vi "_27_Sample_qsns_9[3].vi"() -> ()   [LabVIEW 2020]
panel:
  out "Array":i32[](array[numeric])
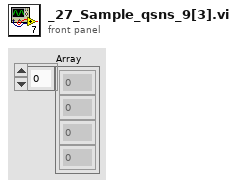
[diagram p1: front panel]
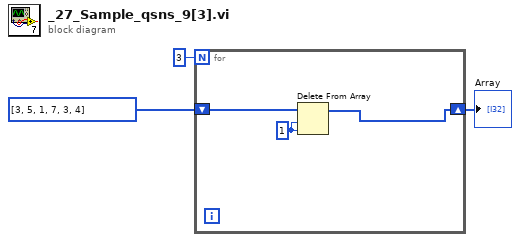
[diagram p0: block diagram]
diagram:
  n1 = for {
    N: 3 -> [_]
    shift-right: [w5] -> w1
    shift-left: i32[] [3, 5, 1, 7, 3, 4] -> [w6]
    w4 = 1 ("index")
    n2 = Delete From Array(array=w6, length=w4, index=w4) -> (array with subset deleted=w5:i32[])  [unwired: 1 out]
  }
  "Array" <- w1
